vi "Target_Distances.vi"(0 "Distance_to_target (in)":dbl) -> (1 "Shooter_RPM_Output":dbl, 2 "Hood_Angle_Output (Deg)":dbl)   [LabVIEW 2019]
uses:
  ArgosLib/ArgosLib.lvlib
panel:
  out "Hood_Angle_Graph":T1(graph)
  out "RPM Graph":cluster{"Distances (in)":dbl[], "RPM":dbl[]}(graph)
  in  "Hood_Angle (Deg)":dbl[](array[numeric])=[63.0, 69.0, 65.0, 61.0]
  in  "RPM":dbl[](array[numeric])=[4000.0, 5000.0, 5000.0, 5000.0]
  in  "Distances (in)":dbl[](array[numeric])=[120.0, 240.0, 360.0, 480.0]
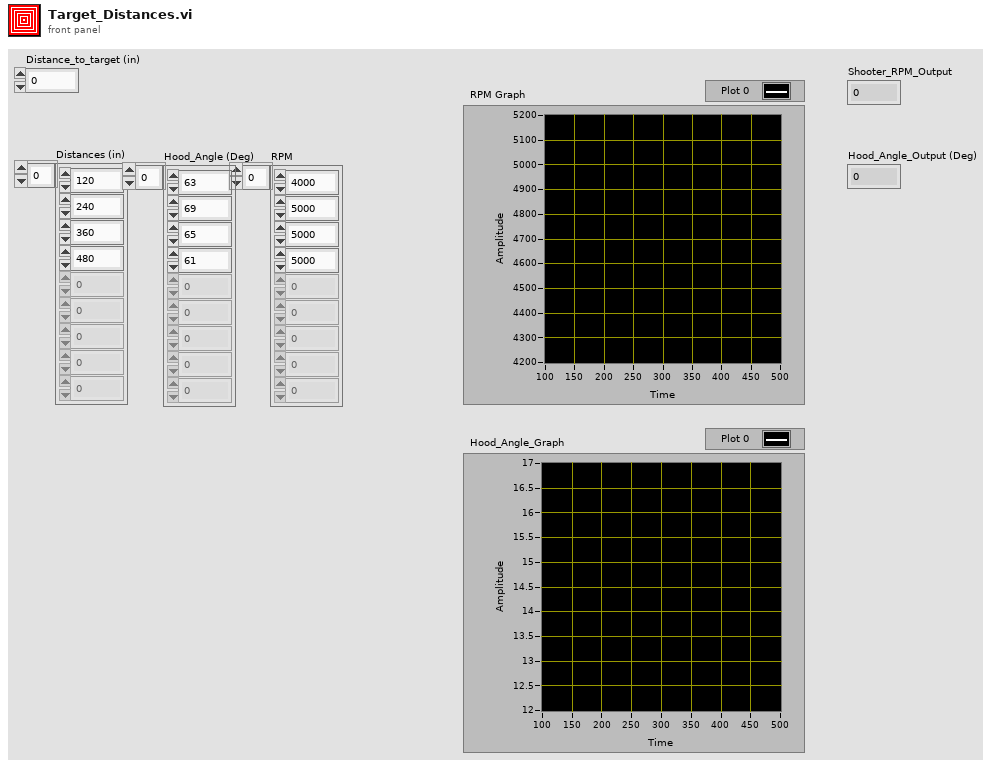
[diagram p1: front panel]
types:
  T1 = cluster{"Distances (in)":dbl[], "Hood_Angle (Deg)":dbl[]}
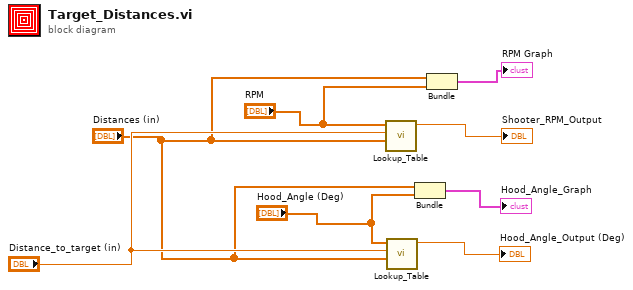
[diagram p0: block diagram]
diagram:
  n1 = call "Lookup_Table.vi"("Y_Array"="RPM", "x_in"="Distance_to_target (in)", "X_Array"="Distances (in)") -> ("y_out"=→"Shooter_RPM_Output":dbl)  [unwired: 6 in]
  n2 = call "Lookup_Table.vi"("Y_Array"="Hood_Angle (Deg)", "x_in"="Distance_to_target (in)", "X_Array"="Distances (in)") -> ("y_out"=→"Hood_Angle_Output (Deg)":dbl)  [unwired: 6 in]
  n3 = Bundle("Distances (in)"="Distances (in)", "Hood_Angle (Deg)"="Hood_Angle (Deg)") -> (→"Hood_Angle_Graph":T1)  [unwired: 1 in]
  n4 = Bundle("Distances (in)"="Distances (in)", "RPM"="RPM") -> (→"RPM Graph":cluster{"Distances (in)":dbl[], "RPM":dbl[]})  [unwired: 1 in]
